vi "Fieldcentric Transform.vi"(7 "X/Y Ratio":dbl, 8 "Gyro Angle":dbl, 10 "Y":dbl, 11 "X":dbl) -> (0 "Robot-rel angle":dbl, 1 "Field-rel angle":dbl, 2 "Vector Y":dbl format="%#_6f", 3 "X Out":dbl)   [LabVIEW 2013]
panel:
  out "XY Graph 2":cluster{dbl[], dbl[]}(graph)
  out "XY Graph":cluster{dbl[], dbl[]}(graph)
  out "Upscaled X":dbl
  out "Actual Ratio Out":dbl
  out "Ratio In":dbl
  out "actual X Power":dbl
  out "Y Out":dbl
  out "Magnitude":dbl
  out "Vector X":dbl format="%#_6f"
  # "<-- should -->\nalways be equal"
  # "OUTPUT ACUTAL POWER"
  # "ROBOT RELATIVE"
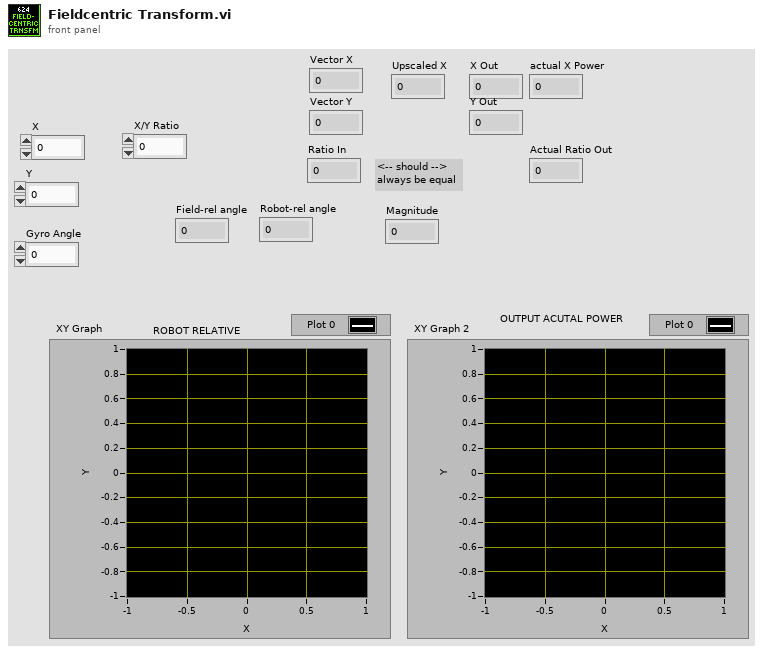
[diagram p1: front panel]
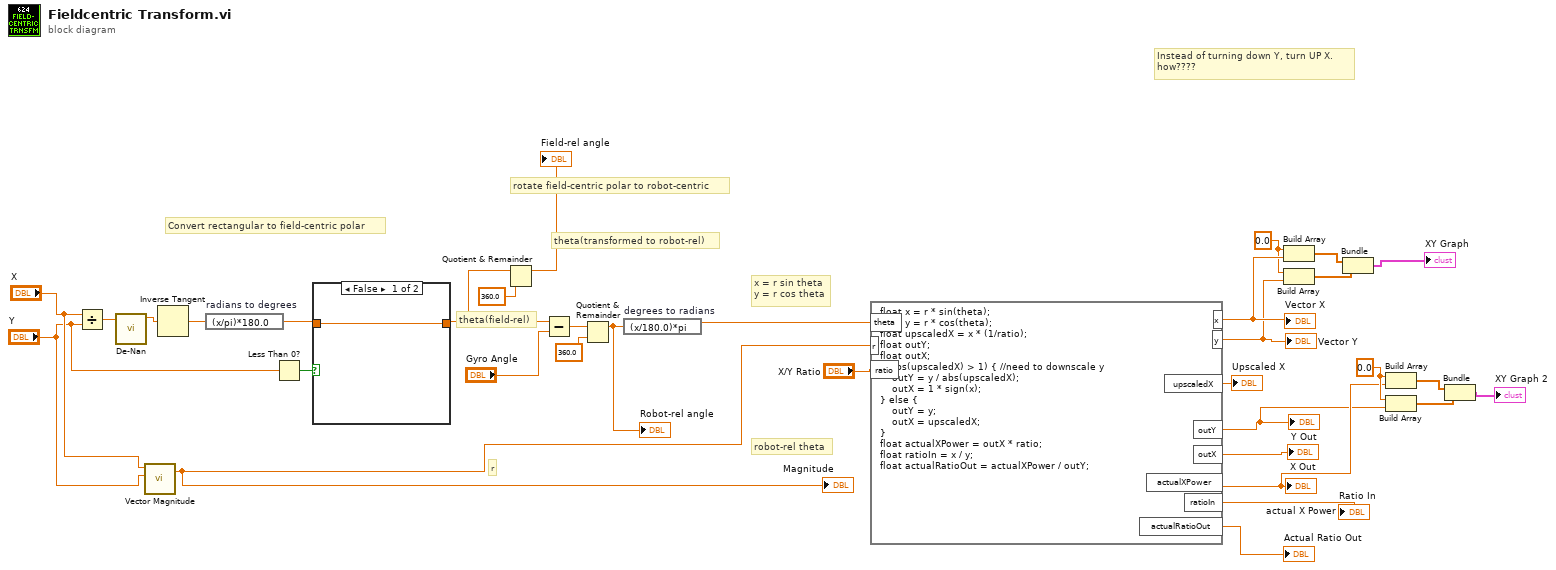
[diagram p0: block diagram]
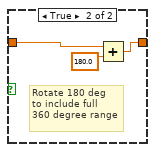
[diagram p2: hidden frame]
diagram:
  w6 = 0.0
  w7 = 0.0
  # "X"
  # "robot-rel theta"
  # "Instead of turning down Y, turn UP X.\nhow????"
  # "theta(field-rel)"
  # "x = r sin theta\ny = r cos theta"
  # "theta(transformed to robot-rel)"
  # "Convert rectangular to field-centric polar"
  # "r"
  # "rotate field-centric polar to robot-centric"
  n1 = Divide(x="X", y="Y") -> (x/y=w23:dbl)
  n2 = call "De-Nan.vi"("output in"=w23) -> ("output out"=w22:dbl)  [unwired: 10 in]
  n3 = call "Vector Magnitude.vi"("Y"="Y", "X"="X") -> ("Magnitude"=w17:dbl)  [unwired: 3 in]
  "Magnitude" <- w17
  n4 = Inverse Tangent(1:w22) -> (0:w30:dbl)
  n5 = expression code="(x/pi)*180.0" "radians to degrees"(w30) -> (w29:dbl)
  n6 = Less Than 0?(x="Y") -> (x < 0?=w33:bool)
  n7 = case shown="False" w33 {
    tunnel: w29 -> [w34 w36]
    tunnel: [w34 w37] -> w25
    frame False {
    }
    frame True {
      # "Rotate 180 deg\nto include full\n360 degree range"
      n8 = Add(x=w36, y=180.0) -> (x+y=w37:dbl)
    }
  }
  n9 = Quotient & Remainder(x=w25, y=360.0) -> (x-y*floor(x/y)=→"Field-rel angle":dbl)  [unwired: 1 out]
  n10 = Subtract(x=w25, y="Gyro Angle") -> (x-y=w32:dbl)
  n11 = Quotient & Remainder(x=w32, y=360.0) -> (x-y*floor(x/y)=w28:dbl)  [unwired: 1 out]
  "Robot-rel angle" <- w28
  n12 = expression code="(x/180.0)*pi" "degrees to radians"(w28) -> (w18:dbl)
  n13 = formula code="float x = r * sin(theta);\nfloat y = r * cos(theta);\nfloat upscaledX = x * (1/ratio);\nfloat outY;\nfloat outX;\nif(abs(upscaledX) > 1) { //need to downscale y\n    outY = y / abs(upscaledX);\n    outX = 1 * sign(x);\n} else {\n    outY = y;\n    outX = upscaledX;\n}\nfloat actualXPower = outX * ratio;\nfloat ratioIn = x / y;\nfloat actualRatioOut = actualXPower / outY;"("theta"=w18, "r"=w17, "ratio"="X/Y Ratio") -> ("outY"=w1:dbl, "outX"=→"X Out":dbl, "x"=w12:dbl, "y"=w11:dbl, "actualXPower"=w2:dbl, "ratioIn"=→"Ratio In":dbl, "actualRatioOut"=→"Actual Ratio Out":dbl, "upscaledX"=→"Upscaled X":dbl)
  "Vector X" <- w12
  "Vector Y" <- w11
  "Y Out" <- w1
  "actual X Power" <- w2
  n14 = Build Array(w7, w12) -> (w9:dbl[])
  n15 = Build Array(w7, w11) -> (w10:dbl[])
  n16 = Bundle(w9, w10) -> (→"XY Graph":cluster{dbl[], dbl[]})  [unwired: 1 in]
  n17 = Build Array(w6, w2) -> (w5:dbl[])
  n18 = Build Array(w6, w1) -> (w4:dbl[])
  n19 = Bundle(w5, w4) -> (→"XY Graph 2":cluster{dbl[], dbl[]})  [unwired: 1 in]
